vi "Read Public Events.vi"(8 "error in (no error)":errorcluster, 11 "Artifactory in":refnum<class "Artifactory.lvclass">) -> (0 "error out":errorcluster, 2 "Public Events":T1, 3 "Artifactory out":refnum<class "Artifactory.lvclass">)   [LabVIEW 2021, in "Artifactory.lvclass"]
uses:
  Artifactory.lvclass
  Artifactory.lvclass/Artifactory.ctl
  Actions -- enum.ctl
  Repository Event -- cluster.ctl
  Public Events -- cluster.ctl
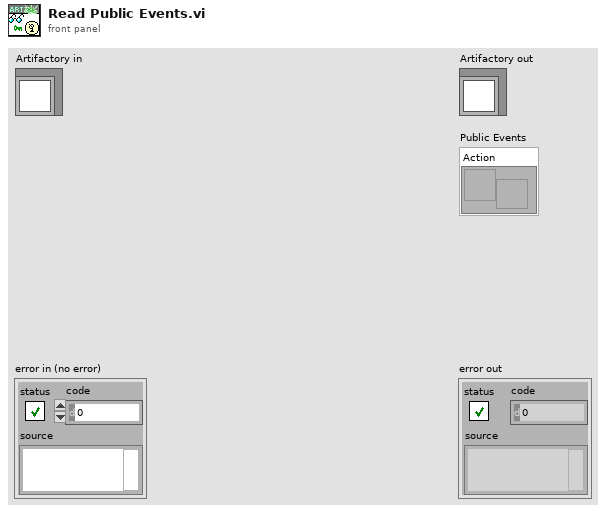
[diagram p1: front panel]
types:
  T1 = typedef "Artifactory.lvclass/Public Events -- cluster.ctl" = cluster{"Action":refnum<user-event>}
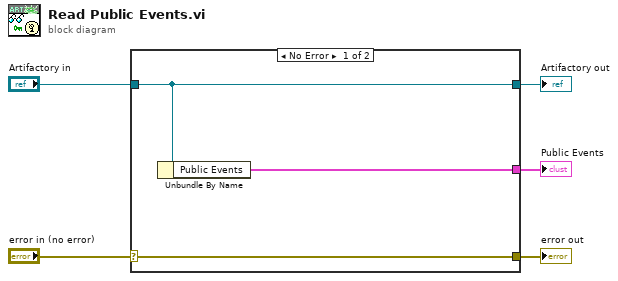
[diagram p0: block diagram]
diagram:
  n1 = case shown="No Error" "error in (no error)" {
    selector: "error in (no error)" -> [w8 w9]
    tunnel: [w8 w9] -> w4
    tunnel: [w7 w10] -> w2
    tunnel: "Artifactory in" -> [w7 w10]
    tunnel: [w6 _] -> w1
    frame No Error {
      n2 = Unbundle By Name(w7) -> ("Public Events"=w6:T1)
    }
    frame Error {
    }
  }
  "error out" <- w4
  "Artifactory out" <- w2
  "Public Events" <- w1
